vi "Set Speed.vi"(8 "error in":errorcluster, 10 "Pump %":dbl, 11 "Masterflex 75211 Settings":T1) -> (0 "error out":errorcluster, 1 "Connection Error":bool, 3 "Masterflex 75211 Settings 2":T1)   [LabVIEW 2018, in "Masterflex 75211.lvlib"]
uses:
  Masterflex 75211.lvlib
  Masterflex 75211 DAQ Setting.ctl
  <vilib>/DAQmx/write.llb/DAQmx Write (Analog DBL 1Chan 1Samp).vi
  <vilib>/DAQmx/write.llb/DAQmx Write (Digital Bool 1Line 1Point).vi
  <vilib>/DAQmx/miscellaneous.llb/DAQmx Fill In Error Info.vi
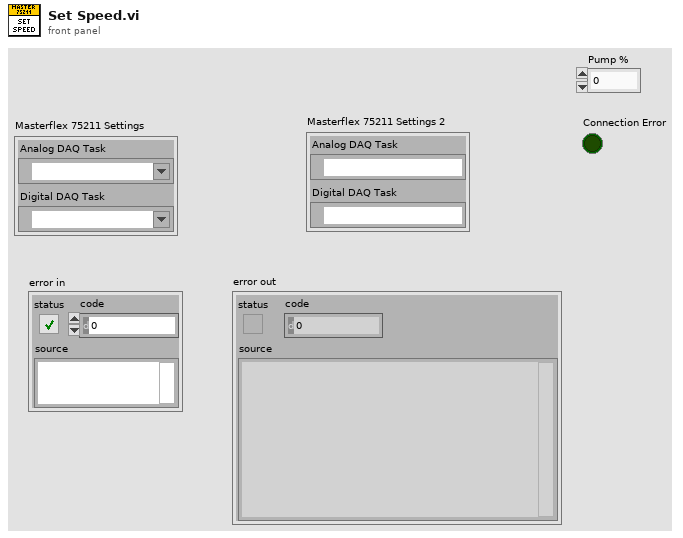
[diagram p1: front panel]
types:
  T1 = typedef "Masterflex 75211.lvlib/Masterflex 75211 DAQ Setting.ctl" = cluster{"Analog DAQ Task":refnum<k21>, "Digital DAQ Task":refnum<k21>}
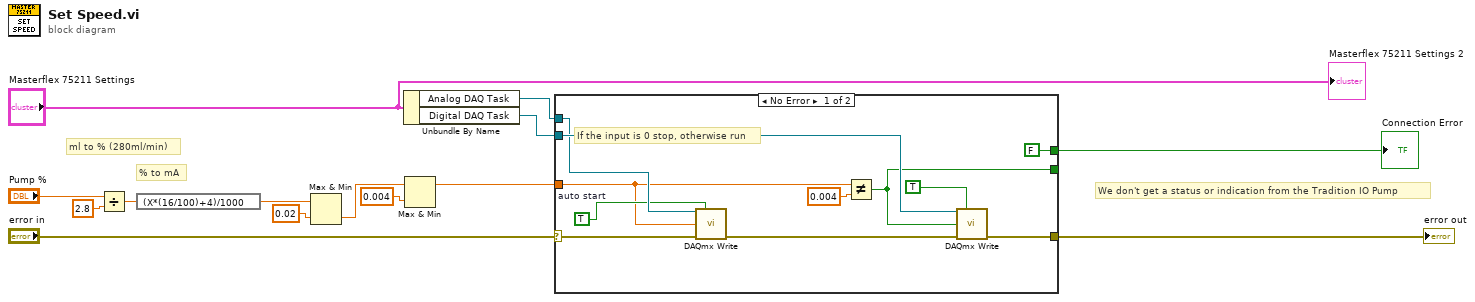
[diagram p0: block diagram]
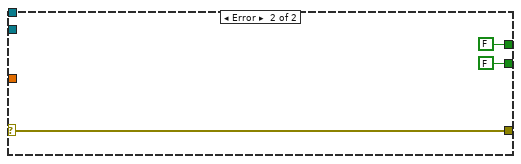
[diagram p2: hidden frame]
diagram:
  # "We don't get a status or indication from the Tradition IO Pump"
  # "ml to % (280ml/min)"
  # "% to mA"
  n1 = Divide(x="Pump %", y=2.8 ("x")) -> (x/y=w9:dbl)
  n2 = expression code="(X*(16/100)+4)/1000"(w9) -> (w5:dbl)
  n3 = Max & Min(x=w5, y=0.02) -> (min(x,y)=w3:dbl)  [unwired: 1 out]
  n4 = Unbundle By Name("Masterflex 75211 Settings") -> ("Analog DAQ Task"=w12:refnum<k21>, "Digital DAQ Task"=w13:refnum<k21>)
  n5 = Max & Min(x=w3, y=0.004) -> (max(x,y)=w1:dbl)  [unwired: 1 out]
  n6 = case shown="No Error" "error in" {
    selector: "error in" -> [w19 w27]
    tunnel: w13 -> [w25 _]
    tunnel: w1 -> [w16 _]
    tunnel: w12 -> [w24 _]
    tunnel: [w20 w27] -> w11
    tunnel: [w17 FALSE ("Pump On?")] -> _
    tunnel: [FALSE ("Connection Error") FALSE ("Connection Error")] -> w8
    frame No Error {
      w22 = TRUE  # auto start
      # "If the input is 0 stop, otherwise run"
      n7 = call-poly <vilib>:"DAQmx Write.vi"("task/channels in"=w24, "auto start"=w22, "data"=w16, "error in"=w19) -> ("error out"=w21:errorcluster)  [unwired: 9 in, 2 out]
      n8 = Not Equal?(x=w16, y=0.004) -> (x != y?=w17:bool)
      n9 = call-poly <vilib>:"DAQmx Write.vi"("task/channels in"=w25, "auto start"=TRUE, "data"=w17, "error in"=w21) -> ("error out"=w20:errorcluster)  [unwired: 9 in, 2 out]
    }
    frame Error {
    }
  }
  "error out" <- w11
  "Connection Error" <- w8
  "Masterflex 75211 Settings 2" <- "Masterflex 75211 Settings"
